vi "sekcje_INI_analog_digital.vi"(11 "section names":string[](array[string])) -> (2 "DI sections":string[](array[string]), 3 "AI sections":string[](array[string]))   [LabVIEW 2013]
doc: "Rozdziela sekcje w pliku ini na\nanalogowe i cyfrowe"
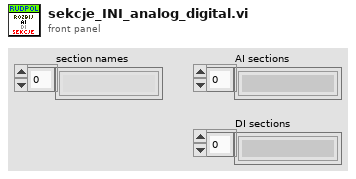
[diagram p1: front panel]
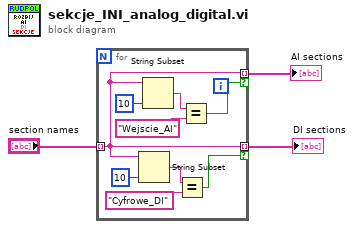
[diagram p0: block diagram]
diagram:
  n1 = for {
    tunnel: "section names" -> [w5] mode=indexing
    tunnel: [w5] -> w3 mode=indexing if=w9
    tunnel: [w5] -> w2 mode=indexing if=w4
    n2 = String Subset(string=w5, length (rest)=10 ("length (rest)")) -> (substring=w7:string)  [unwired: 1 in]
    n3 = String Subset(string=w5, length (rest)=10 ("length (rest)")) -> (substring=w11:string)  [unwired: 1 in]
    n4 = Equal?(x=w7, y="Cyfrowe_DI") -> (x = y?=w4:bool)
    n5 = Equal?(x=w11, y="Wejscie_AI") -> (x = y?=w9:bool)
  }
  "AI sections" <- w3
  "DI sections" <- w2
